vi "Set Sensor Attribute.vi"(8 "error in (no error)":errorcluster caption="错误输入（无错误）", 9 "para2":cluster{} caption="空簇", 10 "attribute":i32, 11 "sensorHandle":i32) -> (0 "error out":errorcluster caption="错误输出", 3 "function return":i32)   [LabVIEW 2018]
doc: "extern int APSxSetSensorAttribute (int sensorHandle, IN int attribute, IN ...);"
uses:
  APSx.dll/APSx.dll
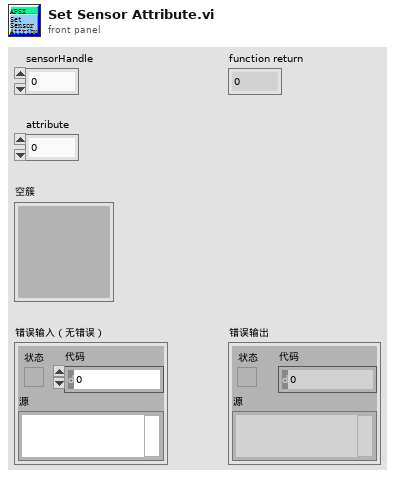
[diagram p1: front panel]
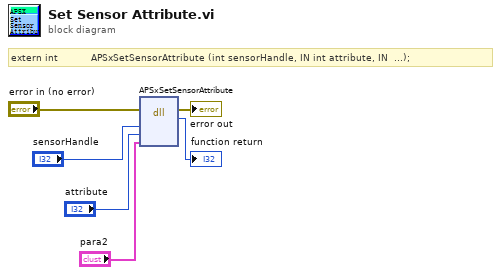
[diagram p0: block diagram]
diagram:
  # "extern int           APSxSetSensorAttribute (int sensorHandle, IN int attribute, IN  ...);"
  n1 = dll-call lib="PTH2[abs D项目Feng恒隆项目Labview传感器对中台SourcesAPSx.dllAPSx.*" fn="APSxSetSensorAttribute"(error in="error in (no error)", "sensorHandle"="sensorHandle", "attribute"="attribute", "para2"="para2") -> (error out=→"error out":errorcluster, "返回类型"=→"function return":i32)  [unwired: 5 in, 1 out]
